vi "SV Remove Delays from Waveforms.vi"   [LabVIEW 2017]
doc: "Use this VI to align waveforms for channels with propagation delay. For each channel, signal delay is added such that all signals have the same (maximum) delay. This common delay is then removed from all signals. This VI maintains a FIFO for each channel to keep the signals aligned with subsequent calls to the VI. The output waveforms will all have the same length. This VI may output waveforms with a different length on reset=TRUE or first call than in subsequent calls."
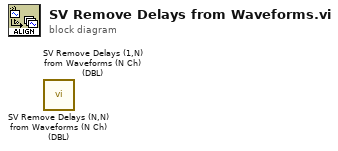
[diagram p0: block diagram]
diagram:
  n1 = call <vilib>:"SV Remove Delays (N,N) from Waveforms (N Ch) (DBL).vi"() -> ()  [unwired: 8 in, 4 out]
  n2 = call <vilib>:"SV Remove Delays (1,N) from Waveforms (N Ch) (DBL).vi"() -> ()  [unwired: 8 in, 4 out]
